vi "Write Selection Color.vi"(6 "Selection Color":u32(colorbox), 11 "File Explorer in":refnum<class "File Explorer.lvclass">) -> (3 "File Explorer out":refnum<class "File Explorer.lvclass">)   [LabVIEW 2017, in "File Explorer.lvlib" / "File Explorer.lvclass"]
uses:
  <vilib>/gpm_packages/@cs/file-explorer-extension/Source/File Explorer/File Explorer/File Explorer.lvclass
  <vilib>/gpm_packages/@cs/file-explorer-extension/Source/File Explorer/File Explorer/File Explorer.lvclass/File Explorer.ctl
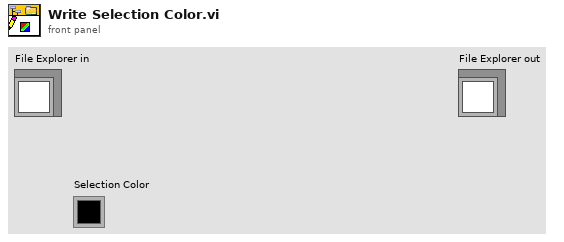
[diagram p1: front panel]
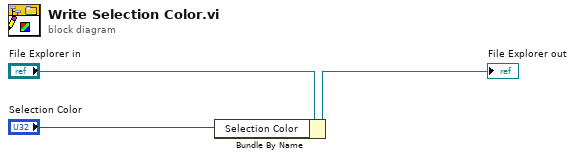
[diagram p0: block diagram]
diagram:
  n1 = Bundle By Name(cluster="File Explorer in", "Selection Color"="Selection Color") -> (→"File Explorer out":refnum<class "File Explorer.lvclass">)
